vi "MultiProcess.vi"(0 "VI Reference In":refnum<vi>, 2 "Label":string, 5 "Wash Array":T1[](array[typedef])=[{"Wash Option"="Underbody Wash", "Car Position"=1, "Elapsed Time"=5.0}, {"Wash Option"="Bug Remover", "Car Position"=1, "Elapsed Time"=5.0}, {"Wash Option"="Pre-Soak", "Car Position"=2, "Elapsed Time"=2.0}, {"Wash Option"="High Pressure Wash", "Car Position"=2, "Elapsed Time"=5.0}, {"Wash Option"="Low Pressure Wax", "Car Position"=2, "Elapsed Time"=5.0}, {"Wash Option"="Spot Free Rinse", "Car Position"=2, "Elapsed Time"=5.0}, {"Wash Option"="Tire Shine Foam", "Car Position"=3, "Elapsed Time"=5.0}, {"Wash Option"="Air Dry", "Car Position"=3, "Elapsed Time"=5.0}], 11 "error in":errorcluster) -> (4 "VI Reference Out":refnum<vi>, 15 "error out":errorcluster)   [LabVIEW 2016]
uses:
  Controls/Wash Step Config.ctl
  main/apis/Stimulus/ValueSignal/ValueSignalByPathString.vi
  main/apis/Stimulus/KeyBoardSimulation/ValueSignalLatchBooleanString.vi
  main/apis/Assert/AssertControlValue/True.vi
  main/Drona.lvlib
  main/apis/Stimulus/ValueSignal/ValueSignal.lvlib
  <vilib>/addons/_JKI Toolkits/Caraya/classes/Test/Test.lvclass
  main/apis/Assert/AssertControlValue/AssertControlValue.lvlib
  main/apis/Stimulus/KeyBoardSimulation/KeyboardSimulation.lvlib
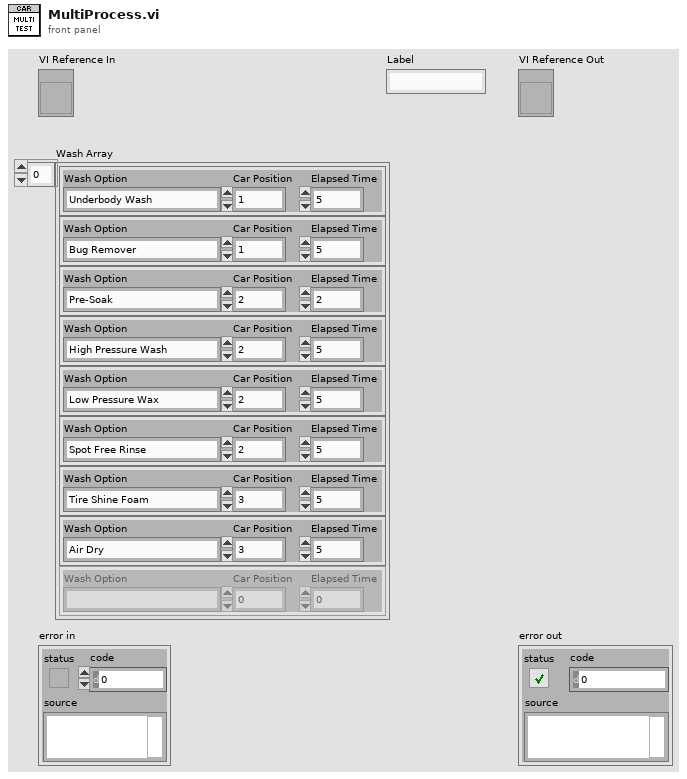
[diagram p1: front panel]
types:
  T1 = typedef "Wash Step Config.ctl" = cluster{"Wash Option":string, "Car Position":u8, "Elapsed Time":dbl}
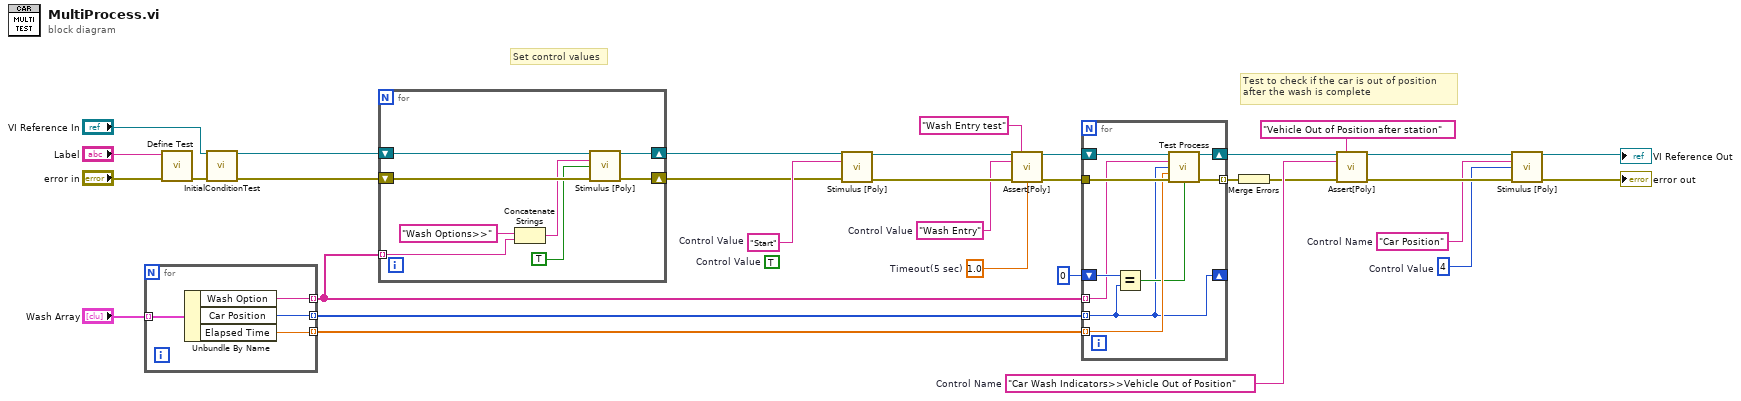
[diagram p0: block diagram]
diagram:
  w25 = "Start"  # Control Value
  (unwired) TRUE  # Control Value
  w16 = u8 4  # Control Value
  w15 = "Car Position"  # Control Name
  w13 = "Car Wash Indicators>>Vehicle Out of Position"  # Control Name
  w12 = 1.0  # Timeout(5 sec)
  w11 = "Wash Entry"  # Control Value
  # "Set control values"
  # "Test to check if the car is out of position \nafter the wash is complete"
  n1 = for {
    tunnel: "Wash Array" -> [w36] mode=indexing
    tunnel: [w35] -> w4 mode=indexing
    tunnel: [w34] -> w6 mode=indexing
    tunnel: [w33] -> w5 mode=indexing
    n2 = Unbundle By Name(w36) -> ("Wash Option"=w35:string, "Car Position"=w34:u8, "Elapsed Time"=w33:dbl)
  }
  n3 = call <vilib>:"Define Test.vi"("error in (no error)"="error in", "Label (VI Title)"="Label") -> ("error out"=w29:errorcluster)  [unwired: 9 in]
  n4 = call "InitialConditionTest.vi"("VI Reference In"="VI Reference In", "error in"=w29) -> ("VI Reference Out"=w32:refnum<vi>, "error out"=w30:errorcluster)  [unwired: 12 in]
  n5 = for {
    tunnel: w4 -> [w42] mode=indexing
    shift-right: [w41] -> w22
    shift-left: w32 -> [w44]
    shift-right: [w40] -> w20
    shift-left: w30 -> [w43]
    n6 = Concatenate Strings("Wash Options>>", w42) -> (w38:string)
    n7 = call-poly "Stimulus [Poly].vi"("VI Reference In"=w44, "Control Path"=w38, "Value (Signaling)"=TRUE, "error in"=w43) -> ("VI Reference Out"=w41:refnum<vi>, "error out"=w40:errorcluster)  [unwired: 10 in]
  }
  n8 = call-poly "Stimulus [Poly].vi"("VI Reference In"=w22, "Control Path"=w25, "error in"=w20) -> ("VI Reference Out"=w24:refnum<vi>, "error out"=w21:errorcluster)  [unwired: 11 in]
  n9 = call-poly "Assert[Poly].vi"("VI Reference In"=w24, "Label"="Wash Entry test", "Control Path"=w11, "Error In"=w21, "Timeout(5 sec)"=w12) -> ("VI Reference Out"=w7:refnum<vi>, "Error Out"=w8:errorcluster)  [unwired: 9 in]
  n10 = for {
    tunnel: w6 -> [w46] mode=indexing
    tunnel: w5 -> [w50] mode=indexing
    shift-right: [w48] -> w3
    shift-left: w7 -> [w51]
    shift-right: [w46] -> _
    shift-left: u8 0 ("Car Position") -> [w53]
    tunnel: w4 -> [w45] mode=indexing
    tunnel: w8 -> [w52]
    tunnel: [w47] -> w2 mode=indexing
    n11 = Equal?(x=w53, y=w46) -> (x = y?=w49:bool)
    n12 = call "Test Process.vi"("VI Reference In"=w51, "Wash Option"=w45, "Car Position"=w46, "Elapsed Time"=w50, "error in"=w52, "Same Position?"=w49) -> ("VI Reference Out"=w48:refnum<vi>, "error out"=w47:errorcluster)  [unwired: 8 in]
  }
  n13 = Merge Errors(w2) -> (w10:errorcluster)
  n14 = call-poly "Assert[Poly].vi"("VI Reference In"=w3, "Label"="Vehicle Out of Position after station", "Control Path"=w13, "Error In"=w10) -> ("VI Reference Out"=w17:refnum<vi>, "Error Out"=w18:errorcluster)  [unwired: 10 in]
  n15 = call-poly "Stimulus [Poly].vi"("VI Reference In"=w17, "Control Path"=w15, "Value (Signaling)"=w16, "error in"=w18) -> ("VI Reference Out"=→"VI Reference Out":refnum<vi>, "error out"=→"error out":errorcluster)  [unwired: 10 in]
